vi "getmessages.vi"(8 "error in (no error)":errorcluster, 11 "hObject":i32) -> (0 "error out":errorcluster, 1 "NumMessages":i32, 2 "pMsgs":T1[](array[typedef]) {"AckBytes [8]" format="%.0x"; "Data [8]" format="%.0x"; "ArbIDOrHeader" format="%.0x"; "DescriptionID" format="%.0x"; "NetworkID" format="%.0x"}, 3 "hObject Out":i32, 4 "NumOfErrors":i32)   [LabVIEW 2009]
doc: "this vi retreives CAN messages from the device. for Non-CAN network, use the \"GetMessages J1850.vi\".\n\n12/21/2010 1.0.0 jyg\n- initial release"
uses:
  ctl spymessage.ctl
  NEO VI Example/data/icsneo40.dll
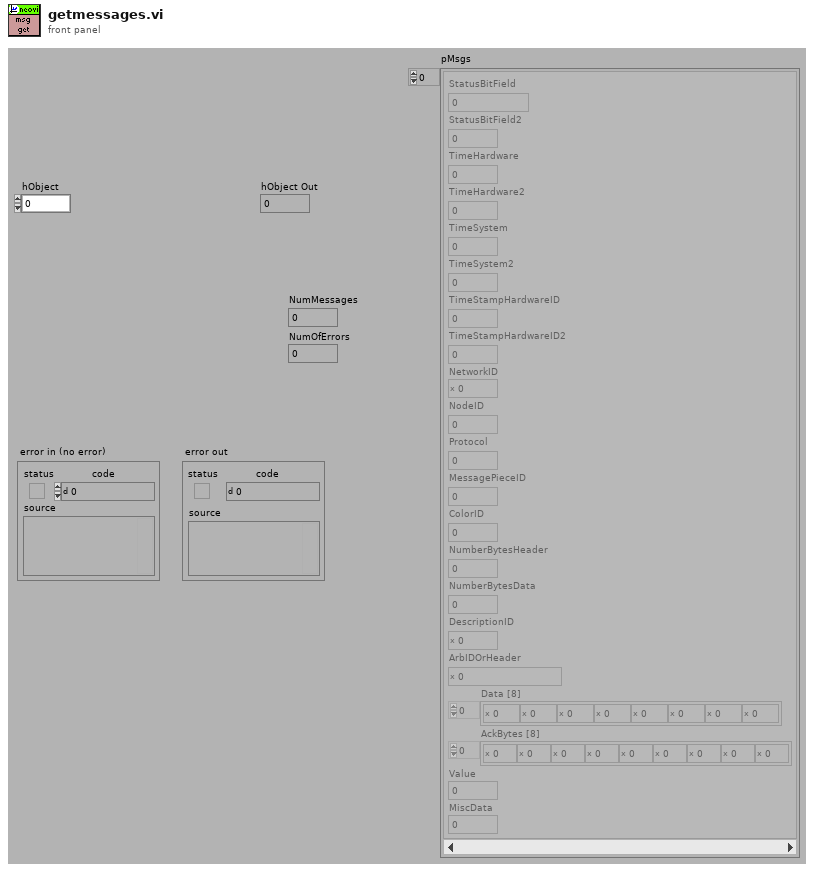
[diagram p1: front panel]
types:
  T1 = typedef "ctl spymessage.ctl" = cluster{"StatusBitField":u32, "StatusBitField2":u32, "TimeHardware":u32, "TimeHardware2":u32, "TimeSystem":u32, "TimeSystem2":u32, "TimeStampHardwareID":u8, "TimeStampHardwareID2":u8, "NetworkID":u8, "NodeID":u8, "Protocol":u8, "MessagePieceID":u8, "ColorID":u8, "NumberBytesHeader":u8, "NumberBytesData":u8, "DescriptionID":u16, "ArbIDOrHeader":u32, "Data [8]":u8[], "AckBytes [8]":u8[], "Value":sgl, "MiscData":u8}
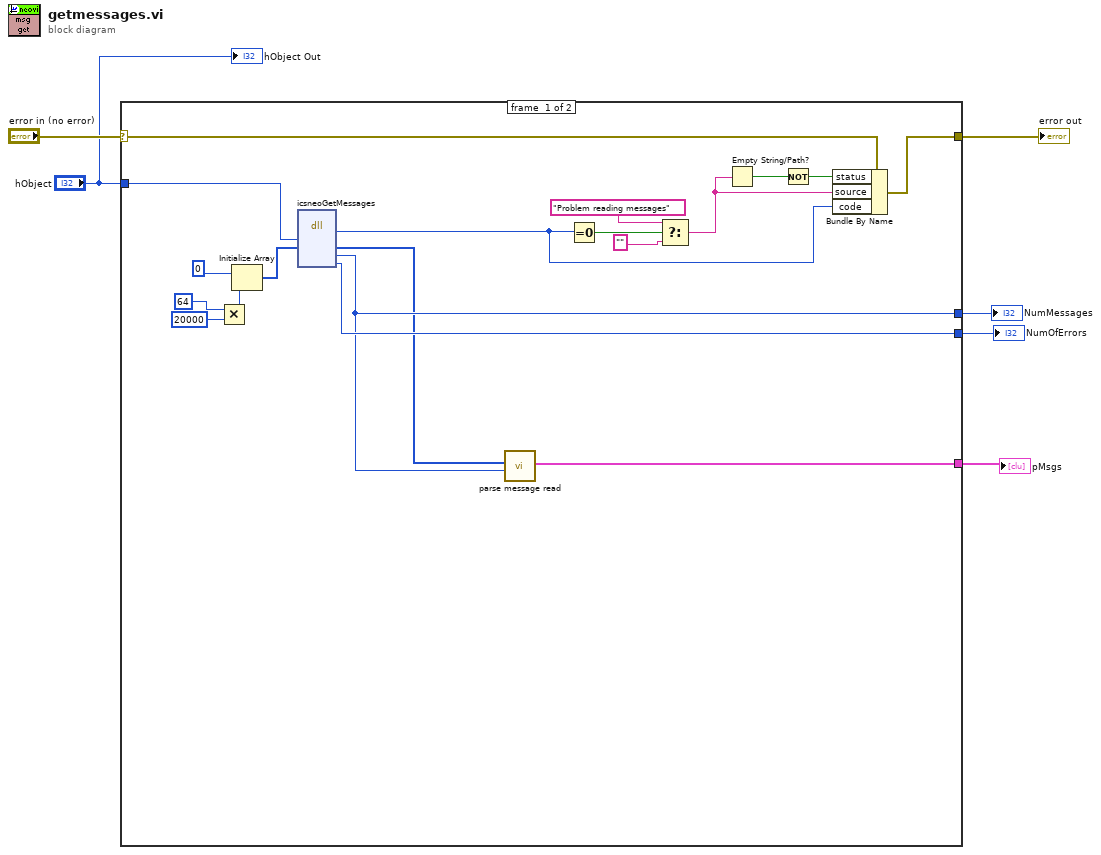
[diagram p0: block diagram]
diagram:
  n1 = case shown="No Error" "error in (no error)" {
    selector: "error in (no error)" -> [w21 w26]
    tunnel: "hObject" -> [w16 _]
    tunnel: [w22 w26] -> w6
    tunnel: [w14 _] -> w3
    tunnel: [w15 _] -> w2
    tunnel: [w7 _] -> w1
    frame #0 {
      n2 = Multiply(x=64 ("dimension size"), y=20000) -> (x*y=w9:i32)
      n3 = Initialize Array(u8 0 ("dimension size"), w9) -> (w10:u8[])
      n4 = dll-call lib="C:/WINDOWS/system32/icsneo40.dll" fn="icsneoGetMessages"("hObject"=w16, "pMsg"=w10) -> ("return type"=w20:i32, "pMsg"=w8:u8[], "pNumberOfMessages"=w14:i32, "pNumberOfErrors"=w15:i32)  [unwired: 4 in, 4 out]
      n5 = call "parse message read.vi"("# of messages"=w14, "Raw Data In"=w8) -> ("Messages out"=w7:T1[])  [unwired: 9 out]
      n6 = Equal To 0?(x=w20) -> (x = 0?=w19:bool)
      n7 = Select(t="Problem reading messages", s=w19, f="") -> (s? t:f=w18:string)
      n8 = Empty String/Path?(string/path=w18) -> (empty?=w24:bool)
      n9 = Not(x=w24) -> (.not. x?=w23:bool)
      n10 = Bundle By Name(cluster=w21, "status"=w23, "source"=w18, "code"=w20) -> (w22:errorcluster)
    }
    frame #1 {
    }
  }
  "error out" <- w6
  "NumMessages" <- w3
  "pMsgs" <- w1
  "NumOfErrors" <- w2
  "hObject Out" <- "hObject"
